vi "Create.vi"(5 "Session (for type)":refnum<class "Session.lvclass">, 8 "error in (no error)":errorcluster, 9 "LabVIEW Version":string, 10 "Source Folder":path) -> (0 "error out":errorcluster, 3 "Session out":refnum<class "Session.lvclass">)   [LabVIEW 2020, in "Save for Previous Version.lvlib" / "Session.lvclass"]
uses:
  Session.lvclass
  Session.lvclass/Session.ctl
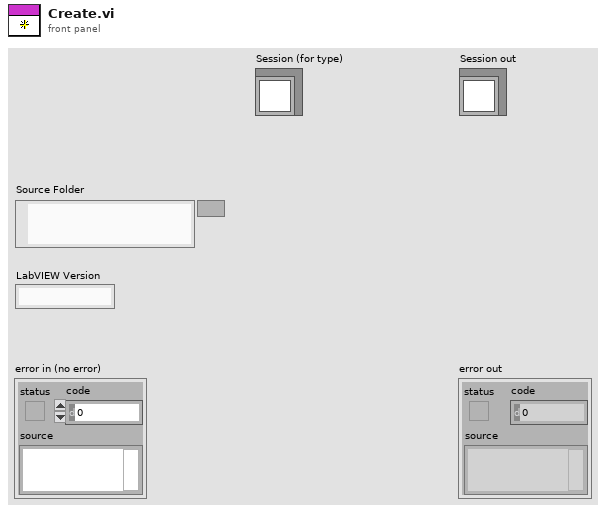
[diagram p1: front panel]
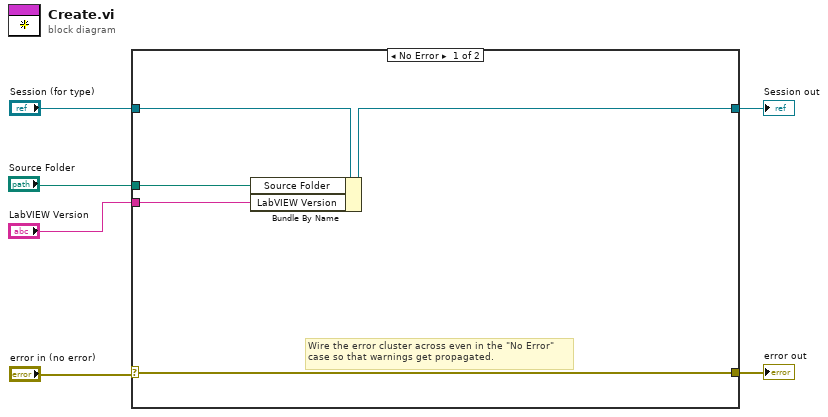
[diagram p0: block diagram]
diagram:
  n1 = case shown="No Error" "error in (no error)" {
    selector: "error in (no error)" -> [w11 w13]
    tunnel: [w11 w13] -> w5
    tunnel: [w8 w12] -> w3
    tunnel: "Session (for type)" -> [w7 w12]
    tunnel: "Source Folder" -> [w10 _]
    tunnel: "LabVIEW Version" -> [w9 _]
    frame No Error {
      # "Wire the error cluster across even in the \"No Error\"\ncase so that warnings get propagated."
      n2 = Bundle By Name(cluster=w7, "Source Folder"=w10, "LabVIEW Version"=w9) -> (w8:refnum<class "Session.lvclass">)
    }
    frame Error {
    }
  }
  "error out" <- w5
  "Session out" <- w3
